vi "solar_app Dir.vi"() -> (1 "solar.ini":path, 2 "AppDir":path, 5 "TempDir?":bool)   [LabVIEW 2018]
doc: "This VI gets the Application Directory and SOLAR.ini path. The AppDir is the *.lvproj or *.exe directory. If neither exist, this returns a temporary path instead."
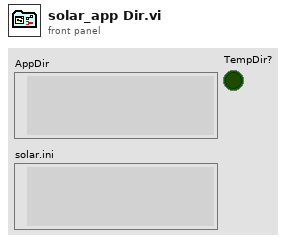
[diagram p1: front panel]
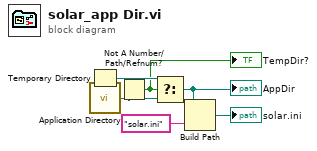
[diagram p0: block diagram]
diagram:
  n1 = Temporary Directory() -> (w2:path)
  n2 = call <vilib>:"Application Directory.vi"() -> ("Application Directory"=w3:path)
  n3 = Not A Number/Path/Refnum?(number/path/refnum=w3) -> (NaN/Path/Refnum?=w1:bool)
  "TempDir?" <- w1
  n4 = Select(t=w2, s=w1, f=w3) -> (s? t:f=w6:path)
  "AppDir" <- w6
  n5 = Build Path(base path=w6, name or relative path="solar.ini") -> (appended path=→"solar.ini":path)
